vi "ShowScanPanel.vi"(6 "SubPanel":refnum<vi>, 8 "error in (no error)":errorcluster caption="entrée d'erreur (pas d'erreur)", 9 "Function":i32, 10 "ScanIndex":i32[][](array[numeric]), 11 "LoadedInst":refnum<class "BaseDevice.lvclass">[](array[class])) -> (0 "sortie d'erreur":errorcluster, 2 "NextPanPos":u32, 3 "LoadedInst Out":refnum<class "BaseDevice.lvclass">[](array[class]) caption="LoadedInst")   [LabVIEW 2019, in "BaseDevice.lvclass"]
uses:
  BaseDevice.lvclass
  BaseDevice.lvclass/BaseDevice.ctl
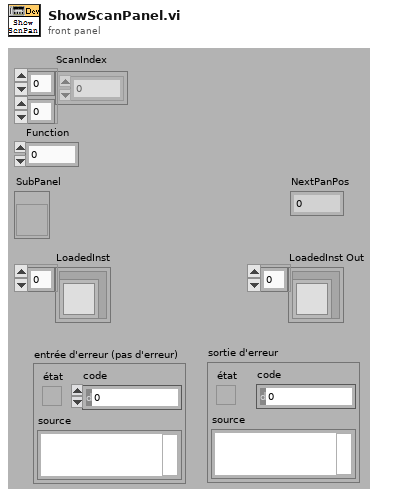
[diagram p1: front panel]
types:
  T1 = typedef "LVPointTypeDef.ctl" = cluster{"Horizontal":i16, "Vertical":i16}
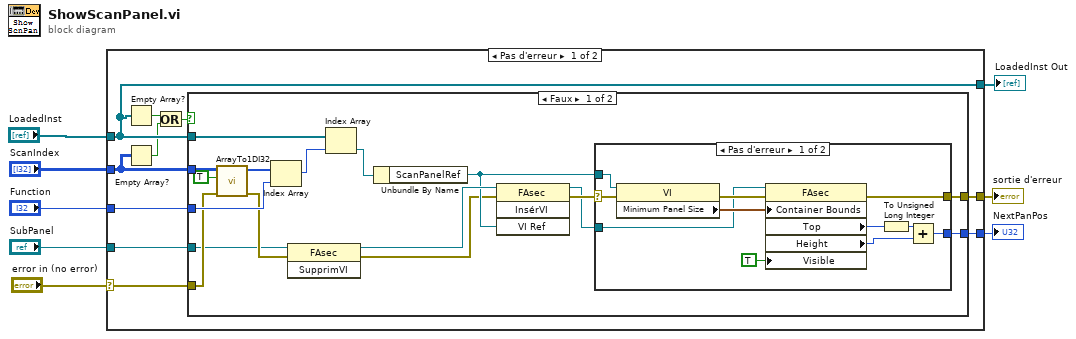
[diagram p0: block diagram]
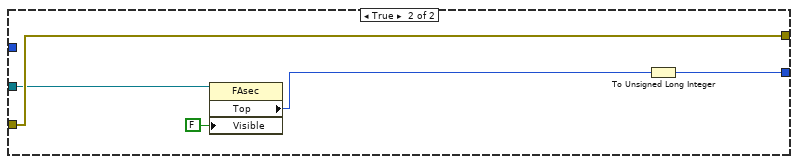
[diagram p3: hidden frame]
diagram:
  n1 = case shown="Pas d'erreur" "error in (no error)" {
    selector: "error in (no error)" -> [w14 w53]
    tunnel: [w16 w53] -> w7
    tunnel: [w13 w54] -> w5
    tunnel: "LoadedInst" -> [w13 w54]
    tunnel: "ScanIndex" -> [w12 _]
    tunnel: "SubPanel" -> [w18 _]
    tunnel: "Function" -> [w17 _]
    tunnel: [w15 _] -> w1
    frame No Error {
      n2 = Empty Array?(array=w13) -> (empty?=w9:bool)
      n3 = Empty Array?(array=w12) -> (empty?=w10:bool)
      n4 = Or(x=w9, y=w10) -> (x .or. y?=w11:bool)
      n5 = case shown="Faux" w11 {
        tunnel: w18 -> [w21 w51]
        tunnel: w17 -> [w33 _]
        tunnel: w13 -> [w31 _]
        tunnel: [w30 w52] -> w16
        tunnel: [w29 w48] -> w15
        tunnel: w12 -> [w28 _]
        tunnel: w14 -> [w26 w52]
        frame False {
          n6 = call <userlib>:"ArrayTo1DI32.vi"("ErrorIn(No Error)"=w26, "DelArrEnd"=TRUE, "tableau"=w28) -> ("sortie d'erreur"=w25:errorcluster, "Array Out"=w27:i32[])  [unwired: 6 in, 1 out]
          n7 = Index Array(array=w27, index=w33) -> (element=w35:i32)
          n8 = invoke on="Nœud de méthode" class="FAsec" method="SupprimVI"(reference=w21, error in=w25) -> (reference out=w34:refnum<vi>, error out=w20:errorcluster)  [unwired: 1 in, 1 out]
          n9 = Index Array(array=w31, index=w35) -> (element=w32:refnum<class "BaseDevice.lvclass">)
          n10 = Unbundle By Name(w32) -> ("ScanPanelRef"=w23:refnum<vi>)
          n11 = invoke on="Nœud de méthode" class="FAsec" method="InsérVI"(reference=w34, error in=w20, "VI Ref"=w23) -> (reference out=w22:refnum<vi>, error out=w24:errorcluster)  [unwired: 1 in, 2 out]
          n12 = case shown="Pas d'erreur" w24 {
            selector: w24 -> [w44 w47]
            tunnel: [w43 w47] -> w30
            tunnel: w23 -> [w41 _]
            tunnel: w22 -> [w40 _]
            tunnel: [w37 _] -> w29
            frame No Error {
              n13 = property class="VI"(reference=w41, error in=w44) -> (error out=w45:errorcluster, "Minimum Panel Size"=w46:T1)  [unwired: 1 out]
              n14 = property class="FAsec"(reference=w40, error in=w45, "Container Bounds"=w46, "Visible"=TRUE) -> (error out=w43:errorcluster, "Top"=w38:i32, "Height"=w39:u32)  [unwired: 1 out]
              n15 = To Unsigned Long Integer(number=w38) -> (unsigned 32bit integer=w36:u32)
              n16 = Add(x=w36, y=w39) -> (x+y=w37:u32)
            }
            frame Error {
            }
          }
        }
        frame True {
          n17 = property class="FAsec"(reference=w51, "Visible"=FALSE) -> ("Top"=w49:i32)  [unwired: 1 in, 2 out]
          n18 = To Unsigned Long Integer(number=w49) -> (unsigned 32bit integer=w48:u32)
        }
      }
    }
    frame Error {
    }
  }
  "sortie d'erreur" <- w7
  "LoadedInst Out" <- w5
  "NextPanPos" <- w1
